vi "Plugin.Initialize.vi"(8 "error in (no error)":errorcluster, 9 "Transceiver":refnum<class "Transceiver.lvclass">, 10 "Transfer Groups":refnum<class "Transfer Group.lvclass">[](array[class]), 11 "Plugin in":refnum<class "Plugin.lvclass">) -> (0 "error out":errorcluster, 3 "Plugin out":refnum<class "Plugin.lvclass">)   [LabVIEW 2017, in "DSF.Engine.lvlib" / "Plugin.lvclass"]
uses:
  Plugin.lvclass
  Transfer/Transfer Group.lvclass
  Transceiver/Transceiver.lvclass
  Plugin.lvclass/Plugin.ctl
  Timing/Timing.lvclass/Timing.ctl
  Debug/Debug Flags.lvclass/Debug Flags.ctl
  Thread Pool/Pool.lvclass/Pool.ctl
  Debug/FIFO Flags.lvclass/FIFO Flags.ctl
  Thread Pool/Pool.Read FIFO.vi
  Thread Pool/Pool.Write FIFO.vi
  Thread Pool/Pool.Get FIFO.vi
  Thread Pool/Pool.Get Debug Flags.vi
  Debug/FIFO Flags.Get Infinite Timeouts.vi
  Thread Pool/ID Pool.lvclass
  C:/Git/DSF/dsf core/Source/Engine/Classes/Thread Pool/Pool.lvclass
  Transceiver/Transceiver Thread.lvclass
  Thread Parameters/Thread Parameters.lvclass
  Timing/Timing.lvclass
  Debug/Debug Flags.lvclass
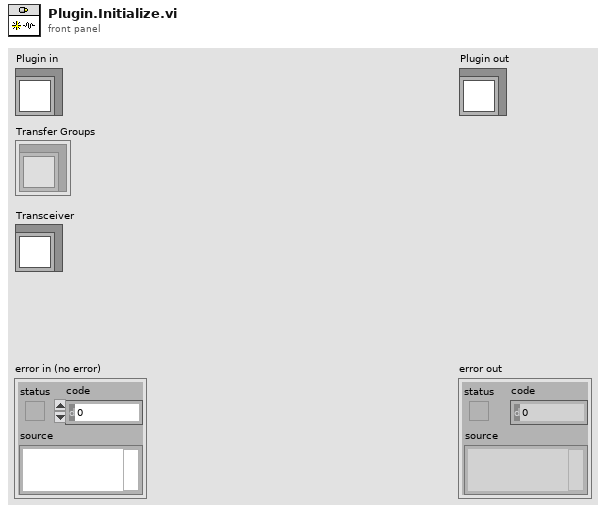
[diagram p1: front panel]
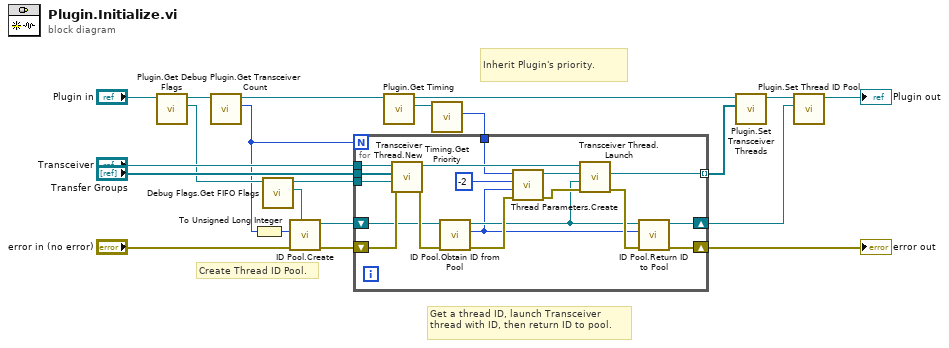
[diagram p0: block diagram]
diagram:
  # "Inherit Plugin's priority."
  # "Get a thread ID, launch Transceiver thread with ID, then return ID to pool."
  # "Create Thread ID Pool."
  n1 = call "Plugin.Get Debug Flags.vi"("Plugin in"="Plugin in") -> ("Debug Flags"=w2:refnum<class "Debug Flags.lvclass">, "Plugin out"=w9:refnum<class "Plugin.lvclass">)  [unwired: 9 in]
  n2 = call "Plugin.Get Transceiver Count.vi"("Plugin in"=w9) -> ("transceiver count"=w1:i32, "Plugin out"=w21:refnum<class "Plugin.lvclass">)  [unwired: 9 in]
  n3 = To Unsigned Long Integer(number=w1) -> (unsigned 32bit integer=w15:u32)
  n4 = call "Debug Flags.Get FIFO Flags.vi"("Debug Flags in"=w2) -> ("FIFO"=w8:refnum<class "FIFO Flags.lvclass">, "Debug Flags out"=w7:refnum<class "Debug Flags.lvclass">)  [unwired: 9 in]
  n5 = call "ID Pool.Create.vi"("FIFO Debug Flags"=w8, "error in (no error)"="error in (no error)", "number of IDs"=w15) -> ("error out"=w6:errorcluster, "ID Pool out"=w16:refnum<class "ID Pool.lvclass">)  [unwired: 7 in]
  n6 = call "Plugin.Get Timing.vi"("Plugin in"=w21) -> ("Timing"=w18:refnum<class "Timing.lvclass">, "Plugin out"=w14:refnum<class "Plugin.lvclass">)  [unwired: 9 in]
  n7 = call "Timing.Get Priority.vi"("Timing in"=w18) -> ("Priority"=w17:u64)  [unwired: 9 in, 1 out]
  n8 = for {
    N: w1 -> [_]
    tunnel: "Transceiver" -> [w39]
    shift-right: [w28] -> w20
    shift-left: w6 -> [w38]
    tunnel: w17 -> [w25]
    tunnel: [w29] -> w13 mode=indexing
    shift-right: [w24] -> w10
    shift-left: w16 -> [w26]
    tunnel: w7 -> [w23]
    tunnel: "Transfer Groups" -> [w22]
    n9 = call "Transceiver Thread.New.vi"("error in (no error)"=w38, "Debug Flags"=w23, "Transfer Groups"=w22, "Transceiver type"=w39) -> ("error out"=w27:errorcluster, "Transceiver Thread out"=w30:refnum<class "Transceiver Thread.lvclass">)  [unwired: 6 in]
    n10 = call "ID Pool.Obtain ID from Pool.vi"("error in (no error)"=w27, "ID Pool in"=w26) -> ("error out"=w36:errorcluster, "id"=w31:i32, "ID Pool out"=w33:refnum<class "ID Pool.lvclass">)  [unwired: 6 in, 1 out]
    n11 = call "Thread Parameters.Create.vi"("error in (no error)"=w36, "id"=w31, "processor"=-2, "priority"=w25) -> ("error out"=w35:errorcluster, "Thread Parameters"=w32:refnum<class "Thread Parameters.lvclass">)  [unwired: 6 in]
    n12 = call "Transceiver Thread.Launch.vi"("error in (no error)"=w35, "Thread ID Pool"=w33, "Thread Parameters"=w32, "Transceiver Thread in"=w30) -> ("error out"=w34:errorcluster, "Interface"=w29:refnum<class "Transceiver Interface.lvclass">)  [unwired: 5 in, 1 out]
    n13 = call "ID Pool.Return ID to Pool.vi"("error in (no error)"=w34, "id"=w31, "ID Pool in"=w33) -> ("error out"=w28:errorcluster, "ID Pool out"=w24:refnum<class "ID Pool.lvclass">)  [unwired: 6 in, 1 out]
  }
  "error out" <- w20
  n14 = call "Plugin.Set Transceiver Threads.vi"("Transceiver Threads"=w13, "Plugin in"=w14) -> ("Plugin out"=w12:refnum<class "Plugin.lvclass">)  [unwired: 9 in]
  n15 = call "Plugin.Set Thread ID Pool.vi"("Thread ID Pool"=w10, "Plugin in"=w12) -> ("Plugin out"=→"Plugin out":refnum<class "Plugin.lvclass">)  [unwired: 9 in]
